vi "Power Accuracy Measurements Key Array.vi"(4 "Conversion":enum16{"Cluster - HTML", "HTML - Cluster"}(ring), 6 "Measurements Key Array In":T4, 7 "Measurements Cluster In":T1 {"Direction" items=["Reverse", "Forward", "Auxiliary"]}) -> (1 "Measurements Cluster Out":T1 {"Direction" items=["Reverse", "Forward", "Auxiliary"]}, 2 "Measurements HTML Out":string)   [LabVIEW 2011]
uses:
  Addons/internet/utils/keyedarr.llb/Keyed Array.ctl
  TypeDefs/Power Accuracy Measurement Parameters.ctl
  SI.LIB/PIM.LIB/HW IO/DUTport.ctl
  SI.LIB/PIM.LIB/HW IO/MeasMode.ctl
  Addons/internet/utils/strutil.llb/Case Matching.ctl
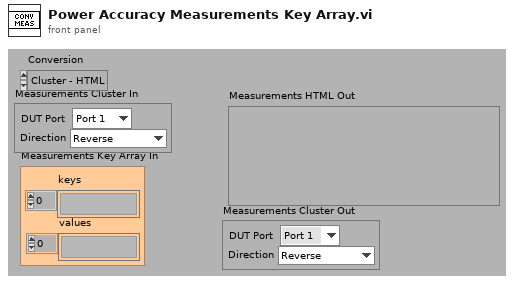
[diagram p1: front panel]
types:
  T1 = typedef "Power Accuracy Measurement Parameters.ctl" = cluster{"DUT Port":T2, "Direction":T3}
  T2 = typedef "DUTport.ctl" = enum16{"Port 1", "Port 2"}
  T3 = typedef "MeasMode.ctl" = u16
  T4 = typedef "Keyed Array.ctl" = cluster{"keys":string[], "values":string[]}
  T5 = typedef "Case Matching.ctl" = enum16{"a != A", "a == A", "system"}
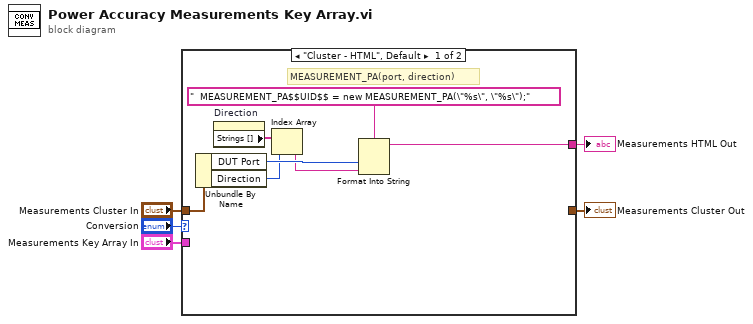
[diagram p0: block diagram]
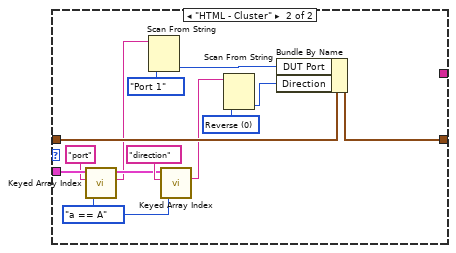
[diagram p2: hidden frame]
diagram:
  n1 = case shown="\"Cluster - HTML\", Default" "Conversion" {
    tunnel: "Measurements Key Array In" -> [_ w25]
    tunnel: "Measurements Cluster In" -> [w12 w23]
    tunnel: [_ w22] -> w3
    tunnel: [w9 _] -> w1
    frame "Cluster - HTML", Default {
      # "MEASUREMENT_PA(port, direction)"
      n2 = Unbundle By Name(w12) -> ("DUT Port"=w10:T2, "Direction"=w8:T3)
      n3 = property on="Direction" class="Ring (strict)"() -> ("Strings []"=w7:string[])  [unwired: 2 in, 2 out]
      n4 = Index Array(array=w7, index=w8) -> (element=w6:string)
      n5 = Format Into String(format string="  MEASUREMENT_PA$$UID$$ = new MEASUREMENT_PA(\"%s\", \"%s\");", w10, w6) -> (resulting string=w9:string)  [unwired: 2 in, 1 out]
    }
    frame "HTML - Cluster" {
      w14 = T3 0 items=["Reverse", "Forward", "Auxiliary"] ("Direction")
      w15 = Case_Matching."a == A" ("case matching (sensitive)")
      n6 = call "Keyed Array Index.vi"("case matching (sensitive)"=w15, "key"="port", "array in"=w25) -> ("value"=w17:string, "duplicate array"=w20:T4)  [unwired: 1 in, 2 out]
      n7 = Scan From String(input string=w17, default 1=DUTport."Port 1" ("Measure.DUT PORT")) -> (output 1=w16:T2)  [unwired: 3 in, 3 out]
      n8 = call "Keyed Array Index.vi"("case matching (sensitive)"=w15, "key"="direction", "array in"=w20) -> ("value"=w19:string)  [unwired: 1 in, 3 out]
      n9 = Scan From String(input string=w19, default 1=w14) -> (output 1=w13:T3)  [unwired: 3 in, 3 out]
      n10 = Bundle By Name(cluster=w23, "DUT Port"=w16, "Direction"=w13) -> (w22:T1)
    }
  }
  "Measurements HTML Out" <- w1
  "Measurements Cluster Out" <- w3
